vi "Tiepie-takeData-2018-06-18.vi"(0 "left rank":i32=2, 1 "right rank":i32=-1, 2 "deBaseline":bool, 3 "Thresh":dbl format="%#_13g", 4 "Laser parameter 2":T2={"VISA resource name"="", "standby"=FALSE, "semaphore in"=refnum, "SetLaserTrans"=0.0, "频率/Hz"=30, "LaserHV"=50} {"LaserHV" min=1 max=100}, 5 "error in (no error)":errorcluster, 7 "ADC parameter":T3) -> (6 "output cluster":cluster{dbl[], "filtered data":dbl[]}, 8 "error out":errorcluster)   [LabVIEW 2013]
uses:
  cal_p.vi
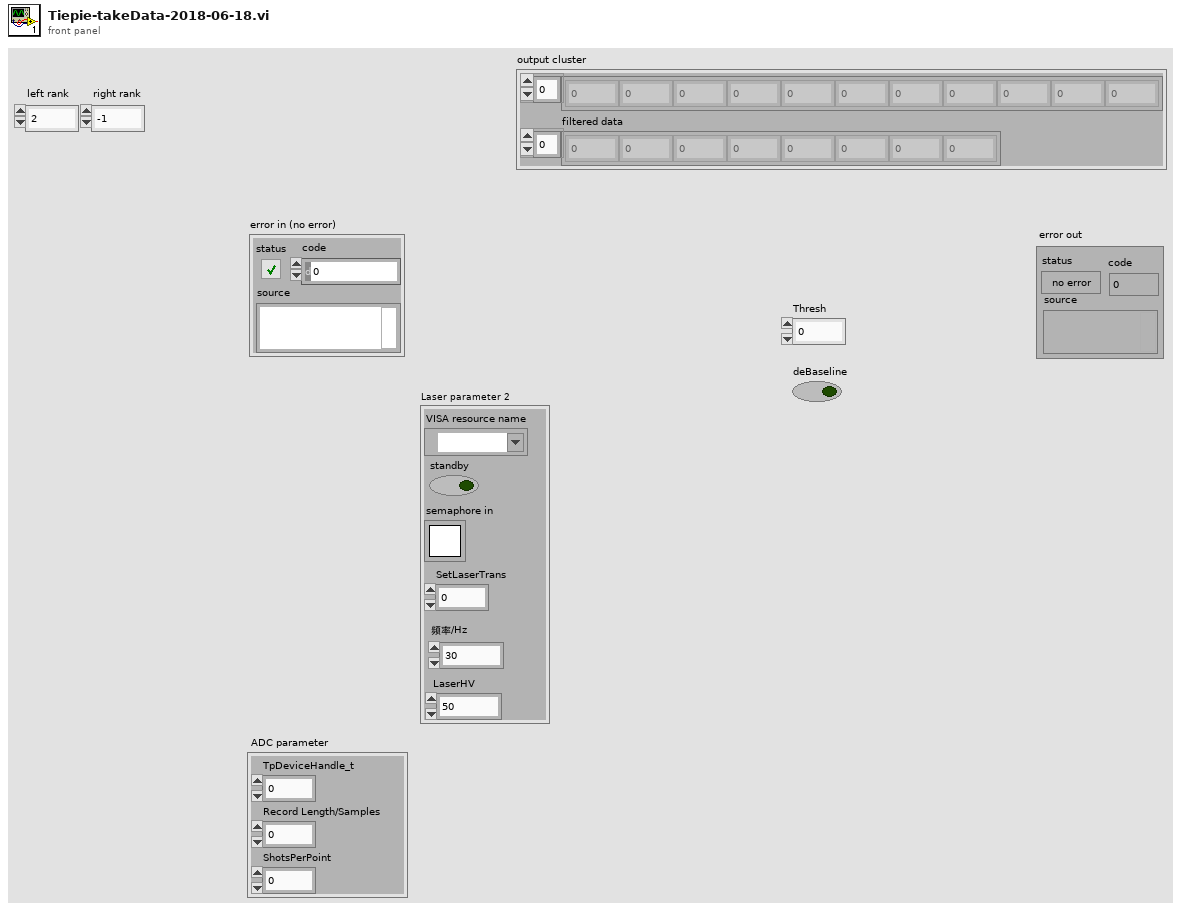
[diagram p1: front panel]
types:
  T1 = typedef "Semaphore RefNum" = refnum<k1>
  T2 = cluster{"VISA resource name":refnum<visa-resource-name>, "standby":bool, "semaphore in":T1, "SetLaserTrans":dbl, "频率/Hz":u8, "LaserHV":u8}
  T3 = cluster{"TpDeviceHandle_t":u32, "Record Length/Samples":u64, "ShotsPerPoint":u16}
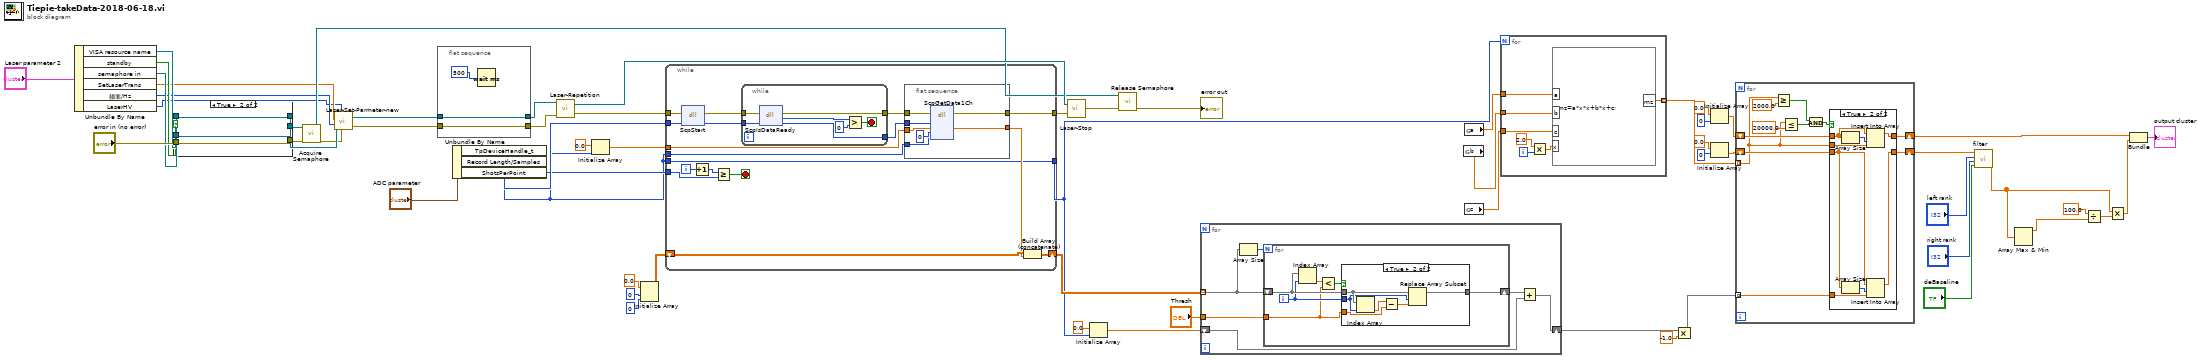
[diagram p0: block diagram]
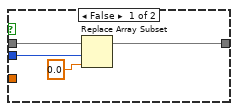
[diagram p3: hidden frame]
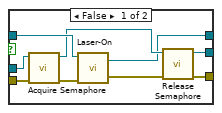
[diagram p4: hidden frame]
diagram:
  n1 = Unbundle By Name("Laser parameter 2") -> ("VISA resource name"=w51:refnum<visa-resource-name>, "standby"=w50:bool, "semaphore in"=w56:T1, "SetLaserTrans"=w9:dbl, "频率/Hz"=w8:u8, "LaserHV"=w7:u8)
  n2 = case shown="True" w50 {
    tunnel: "error in (no error)" -> [w70 w71]
    tunnel: w56 -> [w69 w72]
    tunnel: w51 -> [w66 w73]
    tunnel: [w64 w71] -> w48
    tunnel: [w63 w72] -> w49
    tunnel: [w62 w73] -> w6
    frame False {
      n3 = call <vilib>:"Acquire Semaphore.vi"("error in (no error)"=w70, "semaphore"=w69) -> ("error out"=w68:errorcluster, "semaphore out"=w65:T1)  [unwired: 3 in, 1 out]
      n4 = call "Laser-On.vi"("error in (no error)"=w68, "VISA resource name"=w66) -> ("error out"=w67:errorcluster, "VISA resource name out"=w62:refnum<visa-resource-name>)  [unwired: 2 in]
      n5 = call <vilib>:"Release Semaphore.vi"("error in (no error)"=w67, "semaphore"=w65) -> ("error out"=w64:errorcluster, "semaphore out"=w63:T1)  [unwired: 4 in]
    }
    frame True {
    }
  }
  n6 = call <vilib>:"Acquire Semaphore.vi"("error in (no error)"=w48, "semaphore"=w49) -> ("error out"=w5:errorcluster, "semaphore out"=w36:T1)  [unwired: 3 in, 1 out]
  n7 = call "Laser-Set-Parmeter-new.vi"("error in (no error)"=w5, "LaserHV"=w7, "LaserFreq"=w8, "SetTransmission"=w9, "VISA resource name"=w6) -> ("error out"=w2:errorcluster, "VISA resource name out"=w4:refnum<visa-resource-name>)  [unwired: 1 in]
  n8 = flat-sequence {
    tunnel: w4 -> [w76]
    tunnel: [w76] -> w3
    tunnel: w2 -> [w75]
    tunnel: [w75] -> w1
    frame #0 {
      n9 = Wait (ms)(milliseconds to wait=500) -> ()  [unwired: 1 out]
    }
  }
  n10 = Unbundle By Name("ADC parameter") -> ("TpDeviceHandle_t"=w54:u32, "Record Length/Samples"=w30:u64, "ShotsPerPoint"=w53:u16)
  n11 = call "Laser-Repetition.vi"("error in (no error)"=w1, "VISA resource name"=w3) -> ("error out"=w37:errorcluster, "VISA resource name out"=w47:refnum<visa-resource-name>)  [unwired: 2 in]
  n12 = Initialize Array(0.0, w30) -> (w58:dbl[])
  n13 = Initialize Array(0.0 ("element"), 0 ("dimension size"), 0 ("dimension size")) -> (w60:dbl[][])
  n14 = while {
    tunnel: w54 -> [w93]
    shift-right: [w78] -> w44
    shift-left: w60 -> [w80]
    tunnel: w30 -> [w85]
    tunnel: w58 -> [w84]
    tunnel: w53 -> [w83]
    tunnel: [w82] -> w38
    tunnel: w37 -> [w81]
    tunnel: w30 -> [w77]
    tunnel: [w77] -> w28
    i -> [w90]
    stop <- w86 stop-if-true
    n15 = dll-call lib="PTH1abs CUsers82158Desktop\nä¸æµ·é¡¹ç®2ä¸æµ·é¡¹ç®-2018-05-26ä¸æµ·é¡¹ç®-2018-05-26TOF software\tæ°æ®å¡\nlibtiepie.dll" fn="ScpStart"(error in=w81, "TpDeviceHandle_t"=w93) -> (error out=w92:errorcluster, "TpDeviceHandle_t"=w91:u32)  [unwired: 3 in, 1 out]
    n16 = Increment(x=w90) -> (x+1=w89:i32)
    n17 = Greater Or Equal?(x=w89, y=w83) -> (x >= y?=w86:bool)
    n18 = while {
      tunnel: w92 -> [w107]
      tunnel: w91 -> [w106]
      tunnel: [w105] -> w88
      tunnel: [w104] -> w87
      stop <- w101 stop-if-true
      n19 = dll-call lib="PTH1abs CUsers82158Desktop\nä¸æµ·é¡¹ç®2ä¸æµ·é¡¹ç®-2018-05-26ä¸æµ·é¡¹ç®-2018-05-26TOF software\tæ°æ®å¡\nlibtiepie.dll" fn="ScpIsDataReady"(error in=w107, "TpDeviceHandle_t"=w106) -> (error out=w105:errorcluster, "DataReady"=w102:u8, "TpDeviceHandle_t"=w104:u32)  [unwired: 2 in, 1 out]
      n20 = Greater?(x=w102, y=0 ("index")) -> (0:w101:bool)
    }
    n21 = flat-sequence {
      tunnel: [w100] -> w79
      tunnel: w88 -> [w99]
      tunnel: w87 -> [w98]
      tunnel: w85 -> [w96]
      tunnel: w84 -> [w95]
      tunnel: [w94] -> w82
      frame #0 {
        n22 = dll-call lib="PTH1abs CUsers82158Desktop\nä¸æµ·é¡¹ç®2ä¸æµ·é¡¹ç®-2018-05-26ä¸æµ·é¡¹ç®-2018-05-26TOF software\tæ°æ®å¡\nlibtiepie.dll" fn="ScpGetData1Ch"(error in=w99, "TpDeviceHandle_t"=w98, "pBufferCh1"=w95, "qwStartIndex"=u64 0, "qwSampleCount"=w96) -> (error out=w94:errorcluster, "pBufferCh1"=w100:sgl[])  [unwired: 6 in, 1 out]
      }
    }
    n23 = Build Array (concatenate)(w80, w79) -> (w78:dbl[][])
  }
  n24 = call "Laser-Stop.vi"("error in (no error)"=w38, "VISA resource name"=w47) -> ("error out"=w52:errorcluster)
  n25 = Initialize Array(0.0 ("element"), w28) -> (w42:dbl[])
  n26 = call <vilib>:"Release Semaphore.vi"("error in (no error)"=w52, "semaphore"=w36) -> ("error out"=→"error out":errorcluster)  [unwired: 4 in, 1 out]
  n27 = for {
    tunnel: w44 -> [w113] mode=indexing
    shift-right: [w111] -> w40
    shift-left: w42 -> [w110]
    tunnel: "Thresh" -> [w108]
    n28 = Array Size(array=w113) -> (size(s)=w112:i32)
    n29 = for {
      N: w112 -> [_]
      shift-right: [w117] -> w109
      shift-left: w113 -> [w116]
      tunnel: w108 -> [w114]
      i -> [w115]
      n30 = Index Array(array=w116, index=w115) -> (element=w119:dbl)
      n31 = Less?(x=w119, y=w114) -> (x < y?=w118:bool)
      n32 = case shown="True" w118 {
        tunnel: [w121 w124] -> w117
        tunnel: w116 -> [w123 w129]
        tunnel: w115 -> [w122 w125]
        tunnel: w114 -> [_ w127]
        frame False {
          n33 = Replace Array Subset "Replace Array Subset"(array=w123, new element=0.0 ("new element/subarray"), index=w122) -> (w121:dbl[])
        }
        frame True {
          n34 = Index Array(array=w129, index=w125) -> (element=w128:dbl)
          n35 = Subtract(x=w128, y=w127) -> (x-y=w126:dbl)
          n36 = Replace Array Subset(array=w129, new element=w126, index=w125) -> (w124:dbl[])
        }
      }
    }
    n37 = Add(x=w109, y=w110) -> (x+y=w111:dbl[])
  }
  n38 = global read "cal_p.vi" "b"() -> (w32:dbl)
  n39 = global read "cal_p.vi" "a"() -> (w33:dbl)
  n40 = global read "cal_p.vi" "c"() -> (w31:dbl)
  n41 = for {
    N: w28 -> [_]
    tunnel: [w136] -> w26 mode=indexing
    tunnel: w31 -> [w133]
    tunnel: w32 -> [w134]
    tunnel: w33 -> [w135]
    i -> [w132]
    n42 = Multiply(x=2.0, y=w132) -> (x*y=w130:dbl)
    n43 = formula code="mz=a*x*x+b*x+c;"("a"=w135, "b"=w134, "c"=w133, "x"=w130) -> ("mz"=w136:dbl)
  }
  n44 = Multiply(x=w40, y=-1.0) -> (x*y=w18:dbl[])
  n45 = Initialize Array(0.0 ("element"), 0 ("dimension size")) -> (w21:dbl[])
  n46 = Initialize Array(0.0 ("element"), 0 ("dimension size")) -> (w20:dbl[])
  n47 = for {
    tunnel: w26 -> [w139] mode=indexing
    tunnel: w18 -> [w140] mode=indexing
    shift-right: [w137] -> w16
    shift-left: w20 -> [w141]
    shift-right: [w138] -> w19
    shift-left: w21 -> [w142]
    n48 = Greater Or Equal?(x=w139, y=2000.0) -> (x >= y?=w145:bool)
    n49 = Less Or Equal?(x=w139, y=20000.0) -> (x <= y?=w146:bool)
    n50 = And(x=w145, y=w146) -> (x .and. y?=w143:bool)
    n51 = case shown="True" w143 {
      tunnel: w142 -> [w149 w157]
      tunnel: w141 -> [w148 w156]
      tunnel: w140 -> [_ w153]
      tunnel: w139 -> [_ w152]
      tunnel: [w148 w151] -> w137
      tunnel: [w149 w150] -> w138
      frame False {
      }
      frame True {
        n52 = Array Size(array=w157) -> (size(s)=w154:i32)
        n53 = Array Size(array=w156) -> (size(s)=w155:i32)
        n54 = Insert Into Array(array=w157, index=w154, new element=w152) -> (w150:dbl[])
        n55 = Insert Into Array(array=w156, index=w155, new element=w153) -> (w151:dbl[])
      }
    }
  }
  n56 = call "filter.vi"("deBaseline"="deBaseline", "right rank"="right rank", "left rank"="left rank", "data"=w16) -> ("filtered data"=w12:dbl[])  [unwired: 7 in]
  n57 = Array Max & Min(array=w12) -> (max value=w14:dbl)  [unwired: 3 out]
  n58 = Divide(x=100.0, y=w14) -> (x/y=w13:dbl)
  n59 = Multiply(x=w12, y=w13) -> (x*y=w11:dbl[])
  n60 = Bundle(w19, w11) -> (→"output cluster":cluster{dbl[], dbl[]})  [unwired: 1 in]
